vi "FIR Filter PtByPt.vi"(2 "initialize":bool, 3 "Forward Coefficients":dbl[](array[numeric]), 5 "x":dbl format="%0.2f") -> (0 "error":i32, 1 "Filtered x":dbl format="%0.2f")   [LabVIEW 2020, in "NI_PtbyPt.lvlib"]
doc: "Filters <B>x</B> using the FIR filter specified by <B>Forward Coefficients</B>."
uses:
  NI_PtbyPt.lvlib
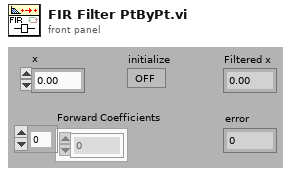
[diagram p1: front panel]
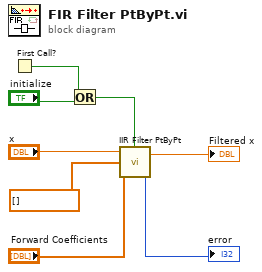
[diagram p0: block diagram]
diagram:
  n1 = First Call?() -> (First Call?: T/F=w1:bool)
  n2 = Or(x=w1, y="initialize") -> (x .or. y?=w3:bool)
  n3 = call "IIR Filter PtByPt.vi"("initialize"=w3, "Forward Coefficients"="Forward Coefficients", "Reverse Coefficients"=dbl[] [], "x"="x") -> ("error"=→"error":i32, "Filtered x"=→"Filtered x":dbl)
